vi "Manual_Inference.vi"() -> ()   [LabVIEW 2023]
uses:
  <vilib>/Platform/TimedLoop/XDataNode/timing_clust.ctl
  <vilib>/Platform/TimedLoop/XDataNode/nitl_modes.ctl
  <vilib>/Platform/TimedLoop/XDataNode/wakeup.ctl
  <vilib>/Analysis/baseanly.llb/Real Dot Product.vi
  <vilib>/platform/TimedLoop/XDataNode/XDataNode.xnode
  <vilib>/Platform/TimedLoop/XDataNode/XDNodeRunTimeDep.lvlib
  <vilib>/Analysis/NI_AALBase.lvlib
panel:
  out "Iter":i32
  in  "stop":bool
  in  "Inputs":dbl[](array[numeric])=[500.0, 200.0, 100.0, 100.0, 200.0, 200.0]
  out "Delta":dbl format="%.2f"
  out "sum":dbl
  out "Outputs":dbl[](array[numeric])
  out "Mean Duration":dbl
  out "Duration Array":i64[](array[numeric])
  out "Sum Duration":i64
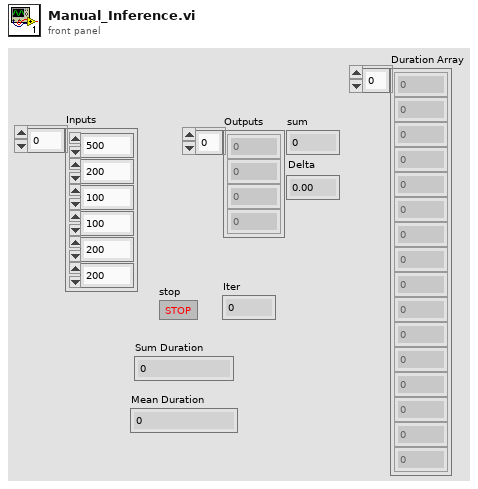
[diagram p1: front panel]
types:
  T1 = typedef "XDNodeRunTimeDep.lvlib/timing_clust.ctl" = cluster{"Expected End [f-1]":u64, "Actual End [f-1]":u64, "Finished Late? [f-1]":bool, "Expected End [i-1]":u64, "Actual End [i-1]":u64, "Finished Late? [i-1]":bool, "Expected Start [i]":u64, "Actual Start [i]":u64, "Expected Start [f]":u64, "Actual Start [f]":u64, "Source Name":string, "Structure Name":string, "Period":i64, "Deadline":i64, "Offset":i64, "Start":i64, "Priority":i32, "Timeout":i32, "Mode":T2, "Wakeup Reason":T3, "Error":errorcluster, "Source Type":string, "Secondary Source Type":string, "Global End Time":u64, "Global Start Time":u64, "Frame Duration":u64, "Iteration Duration":u64, "Assigned CPU":i32, "I/O Scan Engine Mode":u32}
  T2 = typedef "XDNodeRunTimeDep.lvlib/nitl_modes.ctl" = enum32{"No Change", "Process missed periods, maintain original phase", "Discard missed periods, maintain original phase", "Process missed periods, ignore original phase", "Discard missed periods, ignore original phase"}
  T3 = typedef "XDNodeRunTimeDep.lvlib/wakeup.ctl" = enum32{"Normal", "Aborted", "Asynchronous wakeup", "Timing source error", "Timed loop error", "Timeout"}
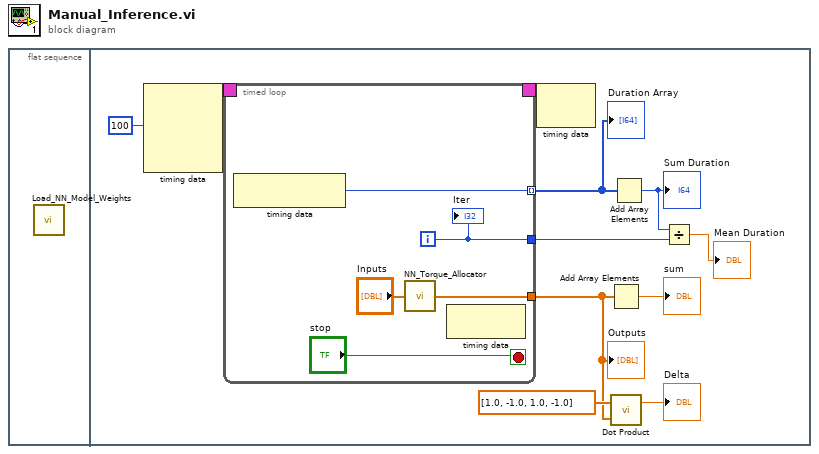
[diagram p0: block diagram]
diagram:
  n1 = flat-sequence {
    frame #0 {
      n2 = call "Load_NN_Model_Weights.vi"() -> ()  [unwired: 12 in]
    }
    frame #1 {
      n3 = node-c288(i64 100 ("Period")) -> (w11:T1)  [unwired: 3 in]
      n4 = timed-loop {
        timing: w11 -> [_]
        timing-out: [_] -> w10
        tunnel: [w16] -> w3 mode=indexing
        tunnel: [w15] -> w2
        tunnel: [w13] -> w1
        i -> [w15]
        stop <- "stop" stop-if-true
        n5 = node-c288() -> (w16:i64)  [unwired: 1 in]
        n6 = call "NN_Torque_Allocator.vi"("Inputs"="Inputs") -> ("Output"=w13:dbl[])
        n7 = node-c288() -> ()  [unwired: 1 in, 1 out]
        "Iter" <- w15
      }
      "Outputs" <- w1
      "Duration Array" <- w3
      n8 = node-c288(w10) -> ()  [unwired: 1 out]
      n9 = Add Array Elements(numeric array=w1) -> (sum=→"sum":dbl)
      n10 = call-poly <vilib>:"Dot Product.vi"("Y Vector"=w1, "X Vector"=dbl[] [1.0, -1.0, 1.0, -1.0]) -> ("X * Y"=→"Delta":dbl)  [unwired: 1 out]
      n11 = Add Array Elements(numeric array=w3) -> (sum=w4:i64)
      "Sum Duration" <- w4
      n12 = Divide(x=w4, y=w2) -> (x/y=→"Mean Duration":dbl)
    }
  }
